vi "TakeMeasurement.vi"(8 "number":dbl, 10 "error in (no error)":errorcluster, 11 "VISA resource name":refnum<visa-resource-name>) -> (0 "Actual_current":dbl caption="Aktuální proud (A)", 1 "Actual_voltage":dbl caption="Aktuální napětí (V)", 2 "error out":errorcluster, 3 "VISA resource output":refnum<visa-resource-name>)   [LabVIEW 2021]
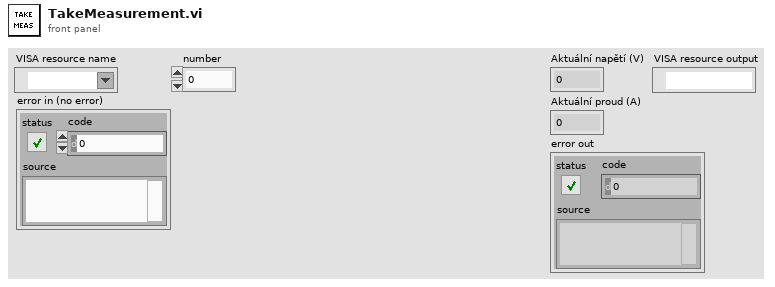
[diagram p1: front panel]
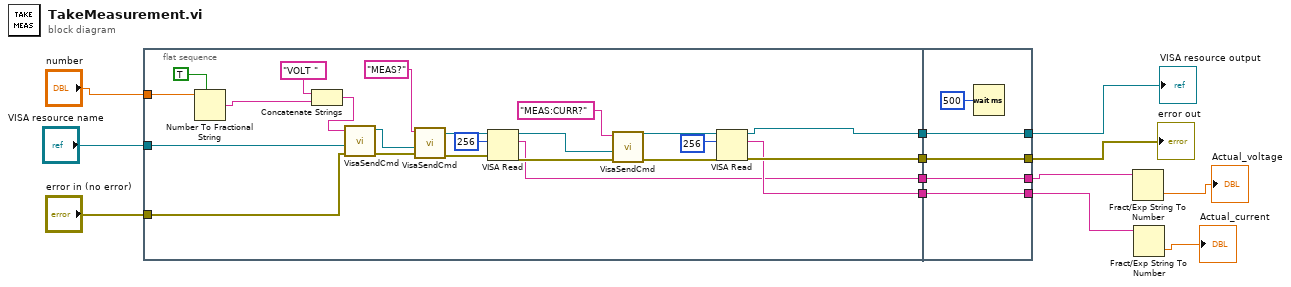
[diagram p0: block diagram]
diagram:
  n1 = flat-sequence {
    tunnel: [w24] -> w13
    tunnel: [w23] -> w12
    tunnel: [w19] -> w11
    tunnel: [w20] -> w10
    tunnel: "VISA resource name" -> [w18]
    tunnel: "error in (no error)" -> [w17]
    tunnel: "number" -> [w14]
    tunnel: w13 -> [w41]
    tunnel: [w41] -> w3
    tunnel: [w40] -> w2
    tunnel: w12 -> [w40]
    tunnel: [w38] -> w6
    tunnel: w11 -> [w38]
    tunnel: w10 -> [w37]
    tunnel: [w37] -> w4
    frame #0 {
      n2 = Number To Fractional String(use system decimal point (T)=TRUE, number=w14) -> (F-format string=w15:string)  [unwired: 2 in]
      n3 = Concatenate Strings("VOLT ", w15) -> (w36:string)
      n4 = call "VisaSendCmd.vi"("error in (no error)"=w17, "VISA resource name"=w18, "Msg to send"=w36) -> ("error out"=w33:errorcluster, "VISA resource output"=w34:refnum<visa-resource-name>)  [unwired: 7 in]
      n5 = call "VisaSendCmd.vi"("error in (no error)"=w33, "VISA resource name"=w34, "Msg to send"="MEAS?") -> ("error out"=w31:errorcluster, "VISA resource output"=w32:refnum<visa-resource-name>)  [unwired: 7 in]
      n6 = VISA Read(VISA resource name=w32, byte count=u32 256, error in (no error)=w31) -> (VISA resource name out=w22:refnum<visa-resource-name>, read buffer=w19:string, error out=w21:errorcluster)  [unwired: 1 out]
      n7 = call "VisaSendCmd.vi"("error in (no error)"=w21, "VISA resource name"=w22, "Msg to send"="MEAS:CURR?") -> ("error out"=w26:errorcluster, "VISA resource output"=w27:refnum<visa-resource-name>)  [unwired: 7 in]
      n8 = VISA Read(VISA resource name=w27, byte count=u32 256, error in (no error)=w26) -> (VISA resource name out=w24:refnum<visa-resource-name>, read buffer=w20:string, error out=w23:errorcluster)  [unwired: 1 out]
    }
    frame #1 {
      n9 = Wait (ms)(milliseconds to wait=u32 500) -> ()  [unwired: 1 out]
    }
  }
  n10 = Fract/Exp String To Number(string=w6) -> (number=→"Actual_voltage":dbl)  [unwired: 3 in, 1 out]
  n11 = Fract/Exp String To Number(string=w4) -> (number=→"Actual_current":dbl)  [unwired: 3 in, 1 out]
  "VISA resource output" <- w3
  "error out" <- w2
